vi "writeToXML.vi"(8 "error in (no error)":errorcluster, 10 "ClassLabel":string, 11 "UpdateIERS in":refnum<class "UpdateIERS.lvclass">) -> (0 "error out":errorcluster, 2 "XML out":string, 3 "UpdateIERS out":refnum<class "UpdateIERS.lvclass">)   [LabVIEW 2022 SP3, in "TCSDataDefinitions.lvlib" / "TCSTimeComponentCommand.lvlib" / "UpdateIERS.lvclass"]
uses:
  UpdateIERS.lvclass
  TCSIersCommand/TCSIersCommand.lvclass
  <userlib>/Common/XML/XMLGenerator/XMLGenerator.lvclass
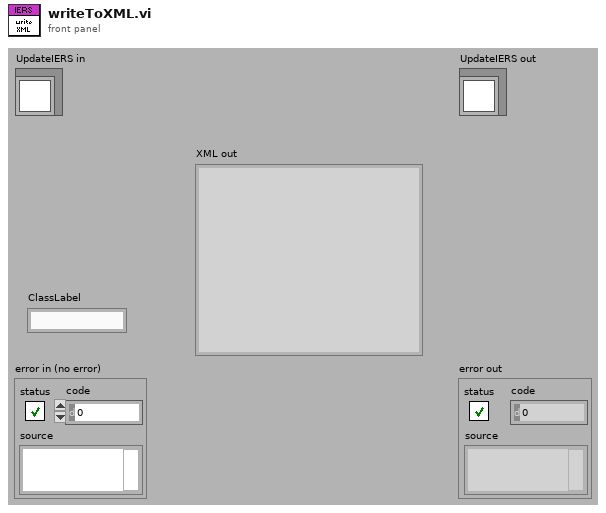
[diagram p1: front panel]
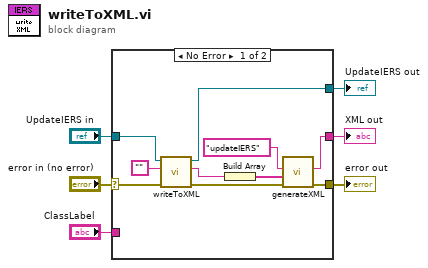
[diagram p0: block diagram]
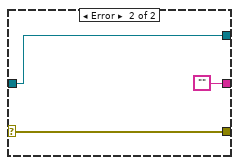
[diagram p2: hidden frame]
diagram:
  n1 = case shown="No Error" "error in (no error)" {
    selector: "error in (no error)" -> [w15 w19]
    tunnel: [w10 w19] -> w5
    tunnel: [w12 w18] -> w3
    tunnel: "UpdateIERS in" -> [w13 w18]
    tunnel: [w9 ""] -> w2
    tunnel: "ClassLabel" -> [_ _]
    frame No Error {
      n2 = call-parent "writeToXML.vi"("error in (no error)"=w15, "ClassLabel"="", "TCSIersCommand in"=w13) -> ("error out"=w11:errorcluster, "XMLout"=w14:string, "TCSIersCommand out"=w12:refnum<class "UpdateIERS.lvclass">)  [unwired: 6 in]
      n3 = Build Array(w14) -> (w8:string[])
      n4 = call <userlib>:"generateXML.vi"("error in"=w11, "childrenXML"=w8, "elementName"="updateIERS" ("Class Label")) -> ("error out"=w10:errorcluster, "XML out"=w9:string)  [unwired: 6 in, 1 out]
    }
    frame Error {
    }
  }
  "error out" <- w5
  "UpdateIERS out" <- w3
  "XML out" <- w2
